vi "GetCtrlRef[].vi"(8 "error in (no error)":errorcluster, 11 "Tab Reference":refnum<vi>) -> (0 "error out":errorcluster, 2 "Page Controls":T1, 3 "All Controls in Tab":T1)   [LabVIEW 2010]
doc: "This VI returns references and names for controls on the tab control.\n\nInputs:\nTab Reference - reference to the tab to scan\nerror in - error input cluster\n\nOutputs:\nPage Controls - (cluster[]) contains the references and names of all pages on the tab. The reference and name arrays are in the same order to allow searching and indexing.\n References - ([eference[]) reference to pages\n Names - (string []) names of pages\nAll controls in Tab - (cluster[]) contains the references and name to all controls on the tab. he reference and name arrays are in the same order to allow searching and indexing.\nerror out - error output cluster"
uses:
  Controls/Shift Registers/TYP_CtrlNameArray.ctl
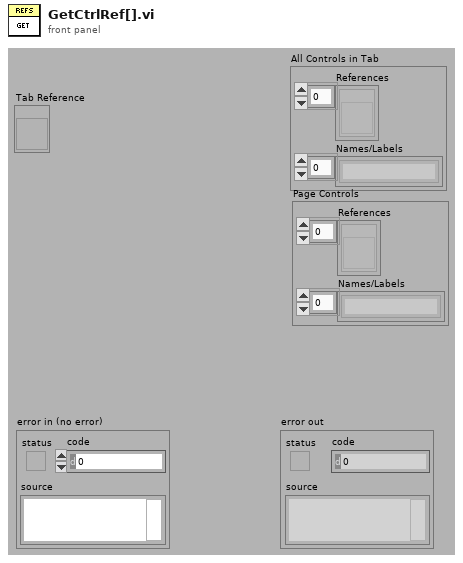
[diagram p1: front panel]
types:
  T1 = typedef "TYP_CtrlNameArray.ctl" = cluster{"References":refnum<vi>[], "Names/Labels":string[]}
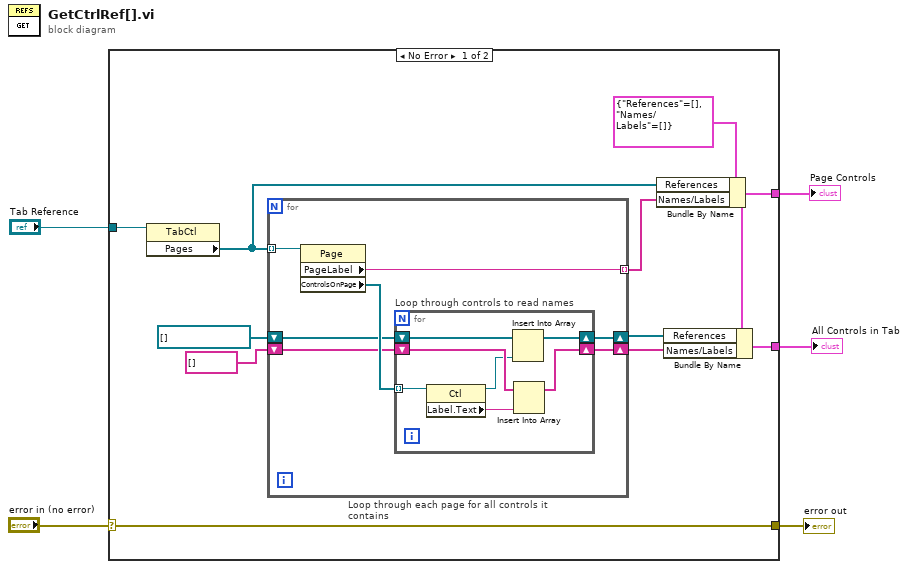
[diagram p0: block diagram]
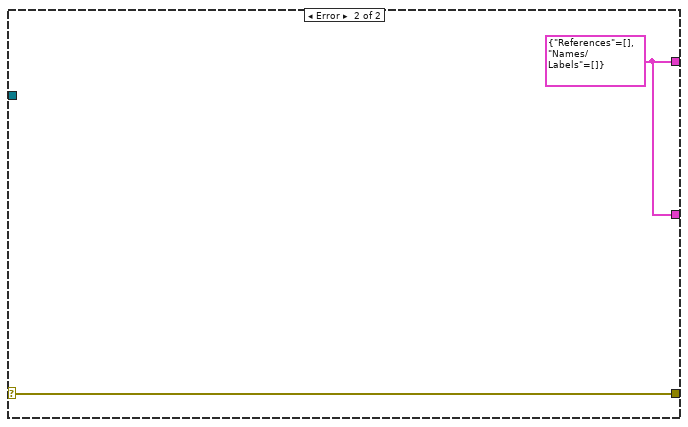
[diagram p2: hidden frame]
diagram:
  n1 = case shown="No Error" "error in (no error)" {
    selector: "error in (no error)" -> [w6 w31]
    tunnel: "Tab Reference" -> [w16 _]
    tunnel: [w15 w32] -> w5
    tunnel: [w13 w32] -> w4
    tunnel: [w6 w31] -> w2
    frame No Error {
      w14 = T1 {"References"=[], "Names/Labels"=[]} ("output cluster")
      n2 = property class="TabCtl"(reference=w16) -> ("Pages"=w12:refnum<vi>[])  [unwired: 1 in, 2 out]
      n3 = for "Loop through each page for all controls it contains" {
        tunnel: w12 -> [w23] mode=indexing
        tunnel: [w22] -> w11 mode=indexing
        shift-right: [w18] -> w7
        shift-left: refnum<vi>[] [] ("Pages") -> [w20]
        shift-right: [w17] -> w8
        shift-left: string[] [] -> [w19]
        n4 = property class="Page"(reference=w23) -> ("PageLabel"=w22:string, "ControlsOnPage"=w21:refnum<vi>[])  [unwired: 1 in, 2 out]
        n5 = for "Loop through controls to read names" {
          tunnel: w21 -> [w30] mode=indexing
          shift-right: [w26] -> w18
          shift-left: w20 -> [w25]
          shift-right: [w27] -> w17
          shift-left: w19 -> [w29]
          n6 = property class="Ctl"(reference=w30) -> (reference out=w24:refnum<vi>, "Label.Text"=w28:string)  [unwired: 1 in, 1 out]
          n7 = Insert Into Array(array=w25, new element=w24) -> (w26:refnum<vi>[])  [unwired: 1 in]
          n8 = Insert Into Array(array=w29, new element=w28) -> (w27:string[])  [unwired: 1 in]
        }
      }
      n9 = Bundle By Name(cluster=w14, "References"=w12, "Names/Labels"=w11) -> (w13:T1)
      n10 = Bundle By Name(cluster=w14, "References"=w7, "Names/Labels"=w8) -> (w15:T1)
    }
    frame Error {
      w32 = T1 {"References"=[], "Names/Labels"=[]} ("output cluster")
    }
  }
  "All Controls in Tab" <- w5
  "Page Controls" <- w4
  "error out" <- w2
